vi "Sort2DArray.vi"(8 "\"Sort on\" Col/Row indx (0)":u32, 9 "Direction (asc)":enum16{"Ascending", "Descending"}(ring), 10 "Sort by (col)":T1(ring), 11 "Array in":string[][](array[string])) -> (1 "Index Out of Range?":bool, 2 "Sort indices":i32[](array[numeric]), 3 "Sorted Array":string[][](array[string]))   [LabVIEW 2013, in "main.lvlib"]
uses:
  main.lvlib
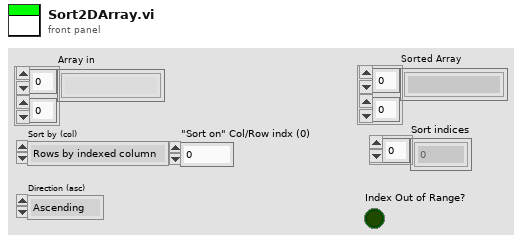
[diagram p1: front panel]
types:
  T1 = enum16{"Rows by indexed column", "Columns by indexed row"}
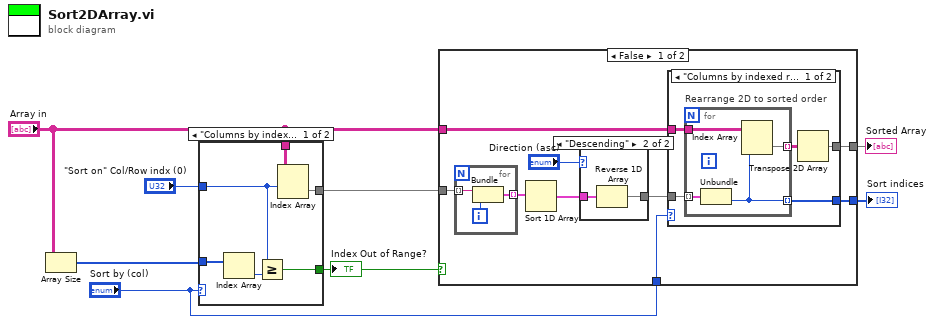
[diagram p0: block diagram]
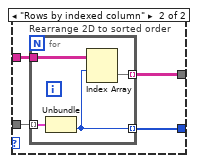
[diagram p2: hidden frame]
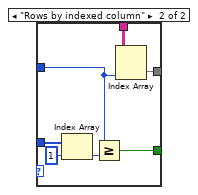
[diagram p5: hidden frame]
diagram:
  n1 = Array Size(array="Array in") -> (size(s)=w4:i32[])
  n2 = case shown="\"Columns by indexed row\"" "Sort by (col)" {
    tunnel: w4 -> [w14 w21]
    tunnel: [w13 w20] -> w3
    tunnel: "\"Sort on\" Col/Row indx (0)" -> [w9 w16]
    tunnel: "Array in" -> [w12 w19]
    tunnel: [w11 w18] -> w6
    frame "Columns by indexed row" {
      n3 = Index Array(array=w14) -> (element=w10:i32)  [unwired: 1 in]
      n4 = Greater Or Equal?(x=w9, y=w10) -> (x >= y?=w13:bool)
      n5 = Index Array(array=w12, index (row)=w9) -> (element=w11:string[])  [unwired: 1 in]
    }
    frame "Rows by indexed column" {
      n6 = Index Array(array=w21, index=1) -> (element=w17:i32)
      n7 = Greater Or Equal?(x=w16, y=w17) -> (x >= y?=w20:bool)
      n8 = Index Array(array=w19, index (col)=w16) -> (element=w18:string[])  [unwired: 1 in]
    }
  }
  "Index Out of Range?" <- w3
  n9 = case shown="False" w3 {
    tunnel: "Array in" -> [w26 w54]
    tunnel: w6 -> [w25 _]
    tunnel: "Sort by (col)" -> [w24 _]
    tunnel: [w23 w54] -> w2
    tunnel: [w22 _] -> w1
    frame False {
      n10 = for {
        tunnel: w25 -> [w49] mode=indexing
        tunnel: [w48] -> w29 mode=indexing
        i -> [w50]
        n11 = Bundle("String"=w49, w50) -> (w48:cluster{"String":string, i32})  [unwired: 1 in]
      }
      n12 = Sort 1D Array(array=w29) -> (sorted array=w28:cluster{"String":string, i32}[])
      n13 = case shown="\"Descending\"" "Direction (asc)" {
        tunnel: [w51 w52] -> w27
        tunnel: w28 -> [w51 w53]
        frame "Ascending", Default {
        }
        frame "Descending" {
          n14 = Reverse 1D Array(array=w53) -> (reversed array=w52:cluster{"String":string, i32}[])
        }
      }
      n15 = case shown="\"Columns by indexed row\"" w24 {
        tunnel: [w32 w43] -> w23
        tunnel: w27 -> [w34 w42]
        tunnel: w26 -> [w33 w41]
        tunnel: [w31 w40] -> w22
        frame "Columns by indexed row" {
          n16 = for "Rearrange 2D to sorted order" {
            tunnel: w34 -> [w39] mode=indexing
            tunnel: w33 -> [w38]
            tunnel: [w37] -> w35 mode=indexing
            tunnel: [w36] -> w31 mode=indexing
            n17 = Unbundle(w39) -> (w36:i32)  [unwired: 1 out]
            n18 = Index Array(array=w38, index (col)=w36) -> (element=w37:string[])  [unwired: 1 in]
          }
          n19 = Transpose 2D Array(2D array=w35) -> (transposed array=w32:string[][])
        }
        frame "Rows by indexed column" {
          n20 = for "Rearrange 2D to sorted order" {
            tunnel: w42 -> [w47] mode=indexing
            tunnel: w41 -> [w46]
            tunnel: [w45] -> w43 mode=indexing
            tunnel: [w44] -> w40 mode=indexing
            n21 = Unbundle(w47) -> (w44:i32)  [unwired: 1 out]
            n22 = Index Array(array=w46, index (row)=w44) -> (element=w45:string[])  [unwired: 1 in]
          }
        }
      }
    }
    frame True {
    }
  }
  "Sorted Array" <- w2
  "Sort indices" <- w1
